vi "Set Dialog Properties.vi"(8 "error in (no error)":errorcluster, 10 "Boolean":bool, 11 "VI in":refnum<vi>) -> (0 "error out":errorcluster)   [LabVIEW 2015]
panel:
  out "VI Ref Out":refnum<vi>
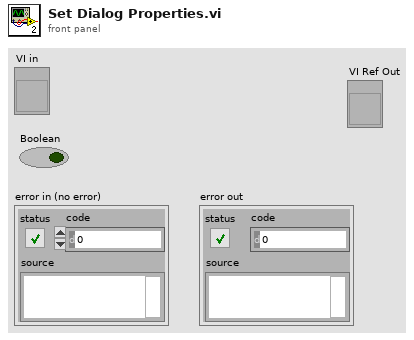
[diagram p1: front panel]
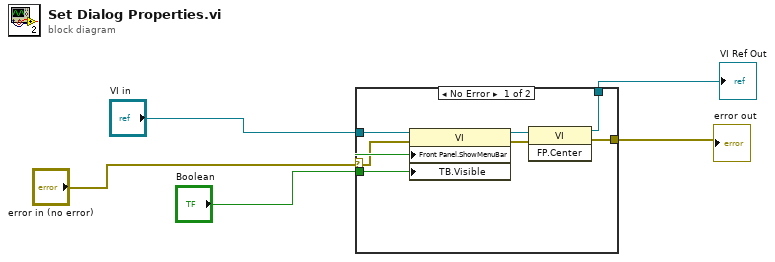
[diagram p0: block diagram]
diagram:
  n1 = case shown="No Error" "error in (no error)" {
    selector: "error in (no error)" -> [w7 w13]
    tunnel: [w12 w13] -> w5
    tunnel: "VI in" -> [w11 w14]
    tunnel: "Boolean" -> [w8 _]
    tunnel: [w6 w14] -> w1
    frame No Error {
      n2 = property class="VI"(reference=w11, error in=w7, "Front Panel.ShowMenuBar"=w8, "TB.Visible"=w8) -> (reference out=w9:refnum<vi>, error out=w10:errorcluster)
      n3 = invoke class="VI" method="FP.Center"(reference=w9, error in=w10) -> (reference out=w6:refnum<vi>, error out=w12:errorcluster)  [unwired: 1 in, 1 out]
    }
    frame Error {
    }
  }
  "error out" <- w5
  "VI Ref Out" <- w1
